vi "set_all_output_types.vi"(8 "error in (no error)":errorcluster, 10 "All output types":string[](array[string]), 11 "VISA resource name":refnum<visa-resource-name>) -> (0 "error out":errorcluster, 3 "VISA resource name out":refnum<visa-resource-name>)   [LabVIEW 2018]
doc: "Update the type of all outputs.\n\nOutputs can normally open or normally closed."
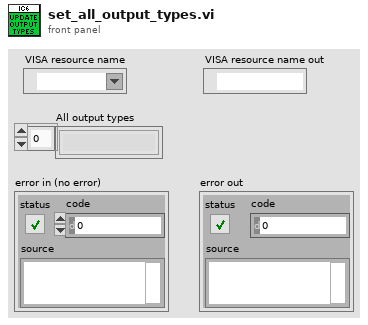
[diagram p1: front panel]
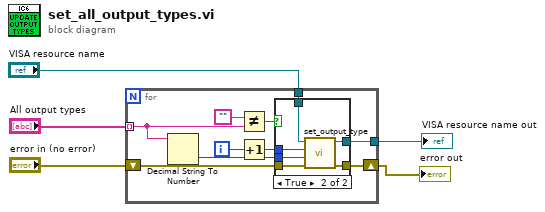
[diagram p0: block diagram]
diagram:
  n1 = for {
    tunnel: "All output types" -> [w7] mode=indexing
    tunnel: "VISA resource name" -> [w11]
    shift-right: [w9] -> w5
    shift-left: "error in (no error)" -> [w10]
    tunnel: [w8] -> w2
    i -> [w15]
    n2 = Decimal String To Number(string=w7) -> (number=w6:i32)  [unwired: 2 in, 1 out]
    n3 = Not Equal?(x="", y=w7) -> (x != y?=w13:bool)
    n4 = Increment(x=w15) -> (x+1=w14:i32)
    n5 = case shown="True" w13 {
      tunnel: w14 -> [_ w23]
      tunnel: w11 -> [w16 w22]
      tunnel: w10 -> [w17 w21]
      tunnel: [w17 w20] -> w9
      tunnel: [w16 w19] -> w8
      tunnel: w6 -> [_ w18]
      frame False {
      }
      frame True {
        n6 = call "set_output_type.vi"("error in (no error)"=w21, "output type"=w18, "output number"=w23, "VISA resource name"=w22) -> ("error out"=w20:errorcluster, "VISA resource name out"=w19:refnum<visa-resource-name>)  [unwired: 6 in]
      }
    }
  }
  "error out" <- w5
  "VISA resource name out" <- w2
